vi "PicoScope4000ExampleAWG.vi"() -> ()   [LabVIEW 2012]
uses:
  ps4000.dll
panel:
  in  "Use Serial Number":bool
  in  "Serial Number":string
  in  "General AWG Settings":T1={"Peak-to-Peak Voltage (microvolts)"=2000000, "Offset Voltage (microvolts)"=0, "Wave Type"=0, "Sweep Type"=0, "Shots"=0, "Sweeps"=0, "Trigger Type"=0, "Trigger Source"=0, "Ext. Threshold (ADC count)"=0, "White Noise/PRBS"=0} {"White Noise/PRBS" items=["Normal", "White Noise", "PRBS"]; "Trigger Source" items=["None", "Scope Trigger", "Aux. In", "Ext. In", "Software Trigger"]; "Trigger Type" items=["Rising", "Falling", "Gate High", "Gate Low"]; "Sweep Type" items=["Up", "Down", "Up-Down", "Down-Up"]; "Wave Type" items=["Sine", "Square", "Triangle", "Ramp Up", "Ramp Down", "Sinc", "Gaussian", "Half Sine", "DC", "White Noise", "Arbitrary"]}
  in  "Arbitrary Waveform Settings":T2 {"Index Mode" items=["Single", "Dual", "Quad"]}
  in  "Standard Waveform Settings":T3={"Start Frequency"=1000.0, "Stop Frequency"=1000.0, "Increment"=0.0, "Dwell Time (seconds)"=0.0} {"Stop Frequency" min=0.03 max=1000000.0; "Start Frequency" min=0.03 max=1000000.0}
  in  "Stop S/W \nTrigger":bool
  in  "Apply Settings":bool
  in  "Stop VI":bool
  in  "Software \nTrigger":bool
  out "Arbitrary\nWaveform Graph":i16[](graph)
  # "If Software trigger is selected, press the 'Stop S/W Trigger'\nbutton prior to selecting 'Apply Settings' or 'Stop VI'."
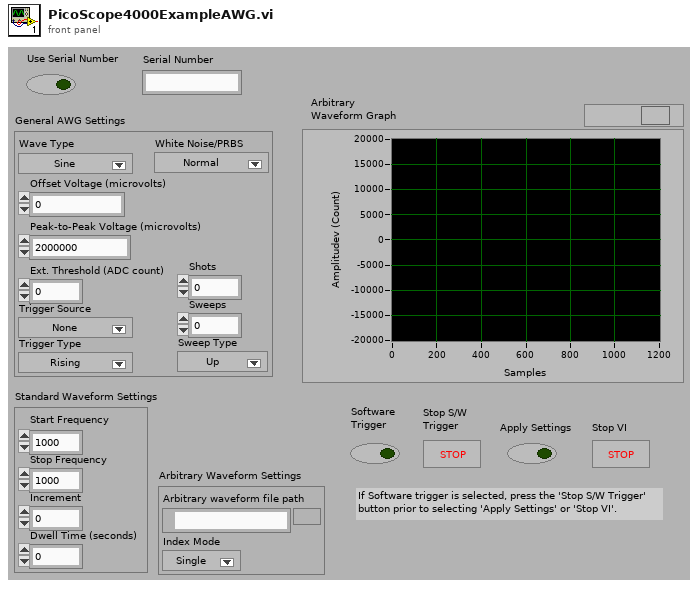
[diagram p1: front panel]
types:
  T1 = cluster{"Peak-to-Peak Voltage (microvolts)":u32, "Offset Voltage (microvolts)":i32, "Wave Type":u32, "Sweep Type":u32, "Shots":u32, "Sweeps":u32, "Trigger Type":u32, "Trigger Source":u32, "Ext. Threshold (ADC count)":i16, "White Noise/PRBS":u32}
  T2 = cluster{"Arbirary waveform file path":path, "Index Mode":u32}
  T3 = cluster{"Start Frequency":dbl, "Stop Frequency":dbl, "Increment":dbl, "Dwell Time (seconds)":dbl}
  T4 = cluster{"Driver Version":string, "USB Version":string, "Hardware":string, "Variant":string, "Batch and Serial":string, "Cal Date":string, "Kernel Version":string, "Num. Channels":i16}
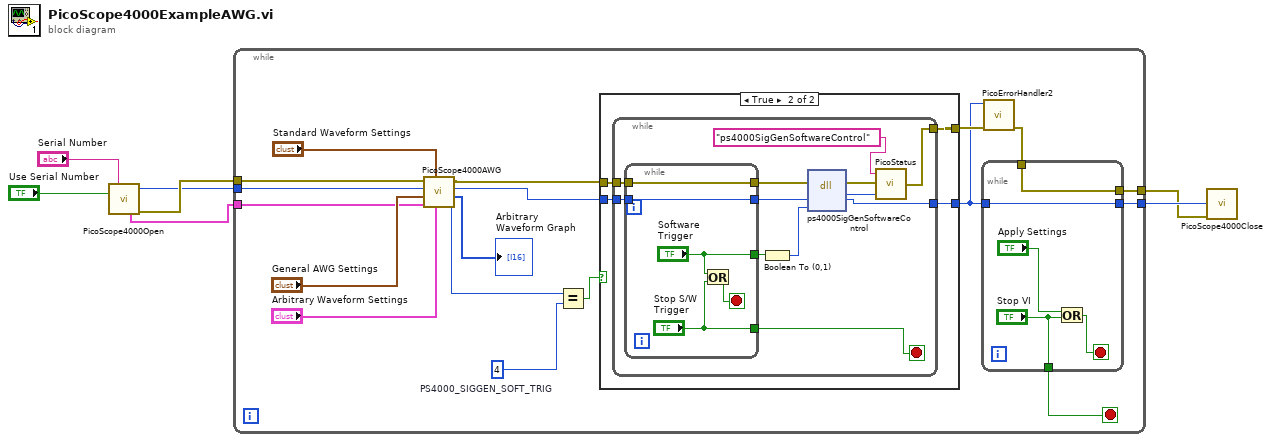
[diagram p0: block diagram]
diagram:
  n1 = call "PicoScope4000Open.vi"("Serial Number"="Serial Number", "Use Serial Number"="Use Serial Number") -> ("handle"=w3:i16, "Unit Info"=w2:T4, "error out"=w4:errorcluster)  [unwired: 10 in, 1 out]
  n2 = while {
    tunnel: w3 -> [w17]
    tunnel: w4 -> [w21]
    tunnel: [w23] -> w7
    tunnel: w2 -> [w12]
    tunnel: [w9] -> w1
    stop <- w22 stop-if-true
    w25 = 4  # PS4000_SIGGEN_SOFT_TRIG
    n3 = call "PicoScope4000AWG.vi"("Arbitrary Waveform Settings"="Arbitrary Waveform Settings", "Standard Waveform Settings"="Standard Waveform Settings", "Unit Info"=w12, "General AWG Settings"="General AWG Settings", "Handle In"=w17, "error in"=w21) -> ("Trigger Source Out"=w16:u32, "Arbitrary\nWaveform Graph"=→"Arbitrary\nWaveform Graph":i16[], "Handle Out"=w18:i16, "error out"=w20:errorcluster)  [unwired: 2 in]
    n4 = Equal?(x=w16, y=w25) -> (x = y?=w24:bool)
    n5 = case shown="True" w24 {
      tunnel: [w32 w33] -> w11
      tunnel: w20 -> [w32 w36]
      tunnel: [w31 w34] -> w10
      tunnel: w18 -> [w31 w35]
      frame False {
      }
      frame True {
        n6 = while {
          tunnel: w36 -> [w47]
          tunnel: w35 -> [w46]
          tunnel: [w44] -> w34
          tunnel: [w39] -> w33
          stop <- w41 stop-if-true
          n7 = while {
            tunnel: [w53] -> w48
            tunnel: w47 -> [w53]
            tunnel: ["Software \nTrigger"] -> w43
            tunnel: w46 -> [w52]
            tunnel: [w52] -> w45
            tunnel: ["Stop S/W \nTrigger"] -> w41
            stop <- w49 stop-if-true
            n8 = Or(x="Software \nTrigger", y="Stop S/W \nTrigger") -> (x .or. y?=w49:bool)
          }
          n9 = Boolean To (0,1)(Boolean=w43) -> (0, 1=w42:i16)
          n10 = dll-call lib="ps4000.dll" fn="ps4000SigGenSoftwareControl"(error in=w48, "handle"=w45, "state"=w42) -> (error out=w40:errorcluster, "PICO_STATUS"=w38:i32, "handle"=w44:i16)  [unwired: 3 in, 1 out]
          n11 = call "PicoStatus.vi"("PICO STATUS"=w38, "error in"=w40, "source"="ps4000SigGenSoftwareControl") -> ("error out"=w39:errorcluster)
        }
      }
    }
    n12 = call "PicoErrorHandler2.vi"("error in (no error)"=w11, "handle In"=w10) -> ("error out"=w8:errorcluster)  [unwired: 9 in]
    n13 = while {
      tunnel: ["Stop VI"] -> w22
      tunnel: [w30] -> w23
      tunnel: w10 -> [w30]
      tunnel: [w26] -> w9
      tunnel: w8 -> [w26]
      stop <- w29 stop-if-true
      n14 = Or(x="Apply Settings", y="Stop VI") -> (x .or. y?=w29:bool)
    }
  }
  n15 = call "PicoScope4000Close.vi"("error in (no error)"=w1, "handle"=w7) -> ()  [unwired: 9 in, 1 out]
